vi "Add Instr CFG.vi"(8 "error in (no error)":errorcluster, 10 "Instr CFG":string, 11 "Configurator JSON Base in":refnum<class "Configurator JSON Base.lvclass">) -> (0 "error out":errorcluster, 3 "Configurator JSON Base out":refnum<class "Configurator JSON Base.lvclass">)   [LabVIEW 2023, in "Configurator JSON Base.lvclass"]
uses:
  Configurator JSON Base.lvclass
  Configurator JSON Base.lvclass/Configurator JSON Base.ctl
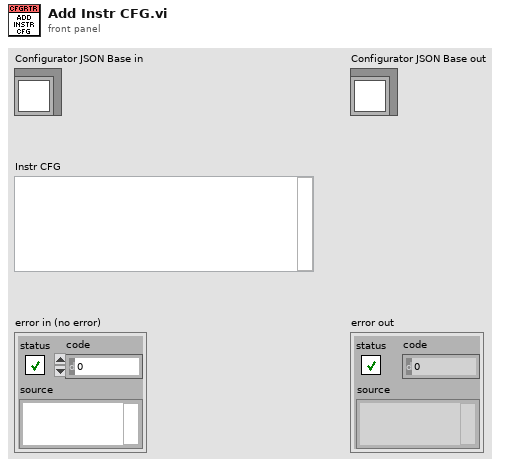
[diagram p1: front panel]
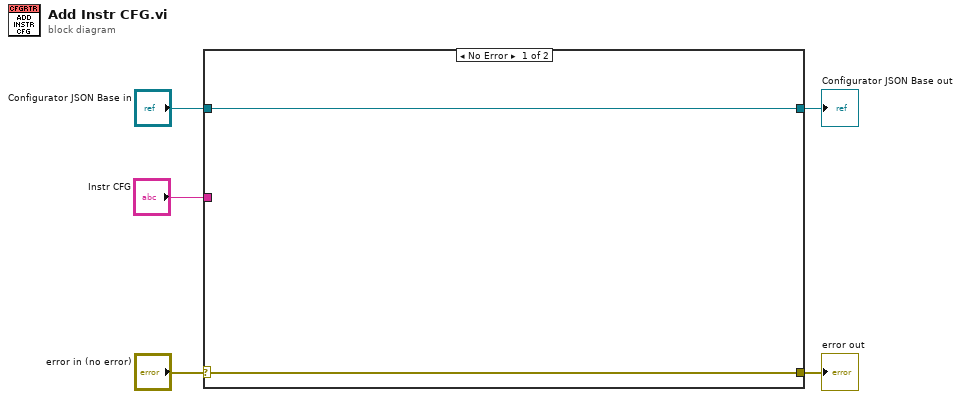
[diagram p0: block diagram]
diagram:
  n1 = case shown="No Error" "error in (no error)" {
    selector: "error in (no error)" -> [w6 w9]
    tunnel: [w6 w9] -> w4
    tunnel: [w7 w8] -> w2
    tunnel: "Configurator JSON Base in" -> [w7 w8]
    tunnel: "Instr CFG" -> [_ _]
    frame No Error {
    }
    frame Error {
    }
  }
  "error out" <- w4
  "Configurator JSON Base out" <- w2
